vi "Startup.vi"(8 "Error In":errorcluster) -> (0 "Error Out":errorcluster)   [LabVIEW 2018]
uses:
  <vilib>/Utility/miscctls.llb/LVPointTypeDef.ctl
  Libraries/Tracker Main/Tracker Main.lvlib
panel:
  in  "Tracker Main to start":bool
  out "Status":string
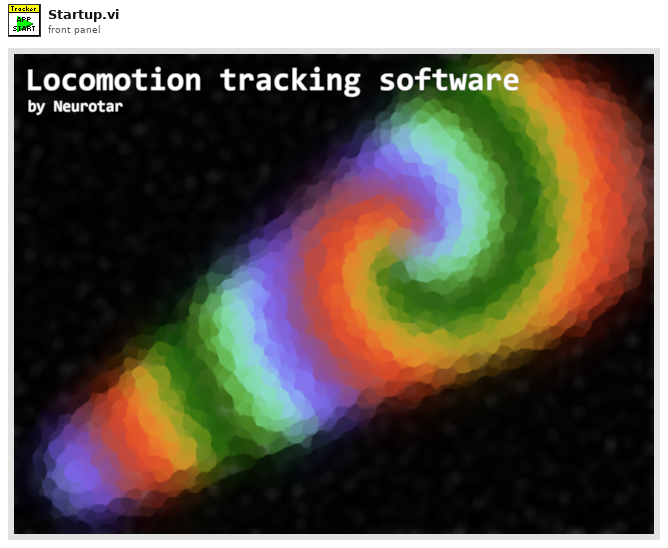
[diagram p1: front panel]
types:
  T1 = typedef "LVPointTypeDef.ctl" = cluster{"Horizontal":i16, "Vertical":i16}
  T2 = enum32{"Invalid", "Standard", "Closed", "Hidden", "Minimized", "Maximized"}
  T3 = typedef "Tracker Main.lvlib/Broadcast Events--cluster.ctl" = cluster{"Module Did Init":refnum<user-event>, "Status Updated":refnum<user-event>, "Error Reported":refnum<user-event>, "Module Did Stop":refnum<user-event>, "Update Module Execution Status":refnum<user-event>}
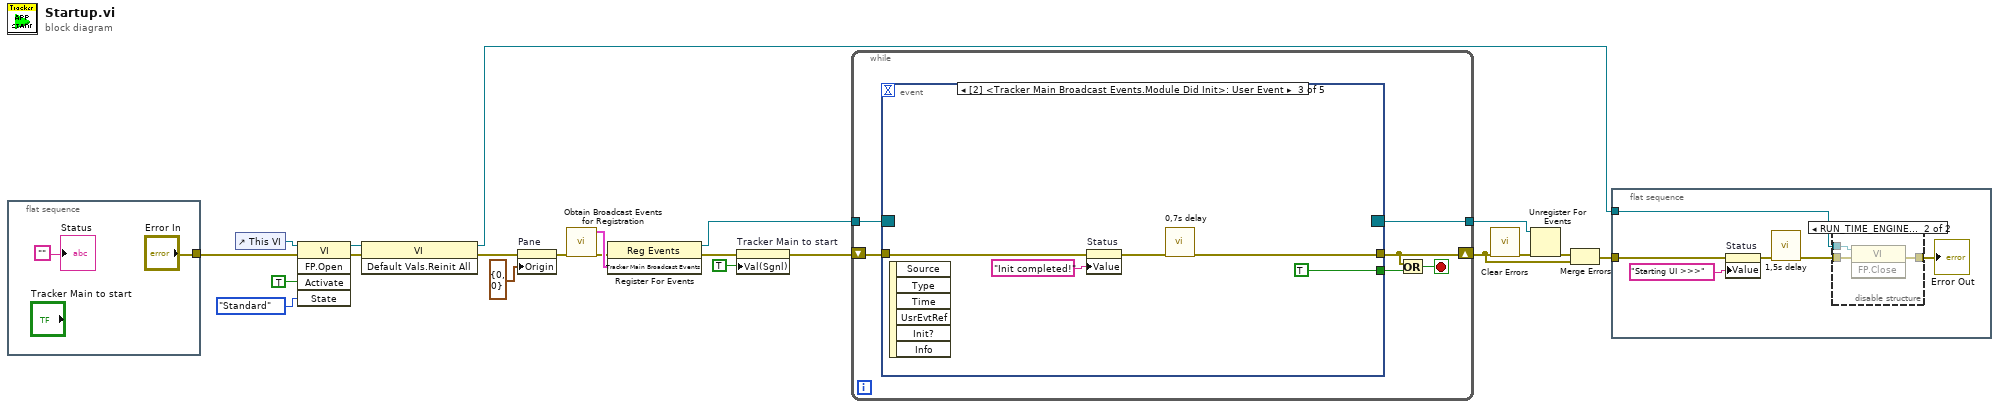
[diagram p0: block diagram]
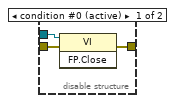
[diagram p2: hidden frame]
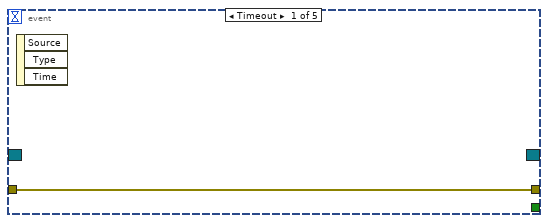
[diagram p3: hidden frame]
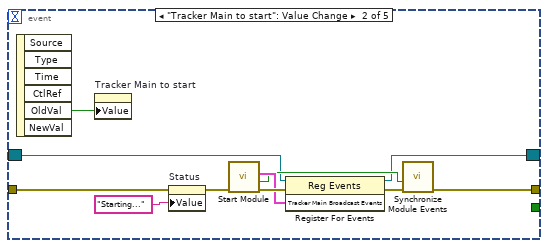
[diagram p4: hidden frame]
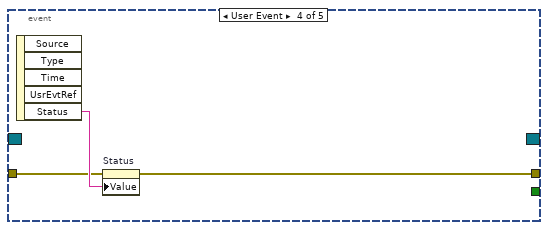
[diagram p5: hidden frame]
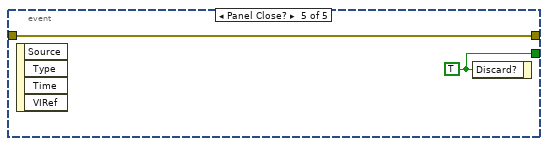
[diagram p6: hidden frame]
diagram:
  n1 = flat-sequence {
    tunnel: ["Error In"] -> w20
    frame #0 {
      "Status" <- ""
    }
  }
  n2 = control-ref of="This VI"() -> (w21:refnum<vi>)
  n3 = invoke class="VI" method="FP.Open"(reference=w21, error in=w20, "Activate"=TRUE ("Activate?"), "State"=T2."Standard") -> (reference out=w16:refnum<vi>, error out=w17:errorcluster)  [unwired: 1 in, 3 out]
  n4 = invoke class="VI" method="Default Vals.Reinit All"(reference=w16, error in=w17) -> (reference out=w1:refnum<vi>, error out=w15:errorcluster)  [unwired: 1 in, 1 out]
  n5 = property on="Pane" class="Pane"(error in=w15, "Origin"=T1 {"Horizontal"=0, "Vertical"=0}) -> (error out=w7:errorcluster)  [unwired: 1 in, 1 out]
  n6 = call "Obtain Broadcast Events for Registration.vi"("error in (no error)"=w7) -> ("error out"=w12:errorcluster, "Tracker Main Broadcast Events"=w13:T3)  [unwired: 8 in, 1 out]
  n7 = register-events(error in=w12, w13) -> (reference out=w11:refnum<event-registration>, error out=w10:errorcluster)  [unwired: 1 in]
  n8 = property on="Tracker Main to start" class="Bool (strict)"(error in=w10, "Val(Sgnl)"=TRUE ("Value (Signaling)")) -> (error out=w9:errorcluster)  [unwired: 1 in, 1 out]
  n9 = while {
    tunnel: w11 -> [w29]
    shift-right: [w25] -> w6
    shift-left: w9 -> [w28]
    tunnel: [w24] -> w3
    stop <- w26 stop-if-true
    n10 = event shown="[2] <Tracker Main Broadcast Events.Module Did Init>: User Event" {
      selector: w29 -> [_ w37 _ _ _]
      dyn-events: [_ w36 _ _ _] -> w24
      timeout: _ -> [_ _ _ _ _]
      tunnel: w28 -> [w30 w32 w45 w48 w50]
      tunnel: [w30 w35 w42 w47 w50] -> w25
      tunnel: [_ _ TRUE _ w51] -> w27
      event Timeout {
        n11 = event-data() -> ()  [unwired: 1 in, 3 out]
      }
      event "Tracker Main to start": Value Change {
        n12 = event-data() -> ("OldVal"=w34:bool)  [unwired: 1 in, 5 out]
        n13 = property on="Tracker Main to start" class="Bool (strict)"("Value"=w34) -> ()  [unwired: 2 in, 2 out]
        n14 = property on="Status" class="Str"(error in=w32, "Value"="Starting..." ("Status")) -> (error out=w31:errorcluster)  [unwired: 1 in, 1 out]
        n15 = call "Start Module.vi"("error in (no error)"=w31) -> ("error out"=w41:errorcluster, "Wait for Event Sync?"=w38:bool, "Tracker Main Broadcast Events"=w40:T3)  [unwired: 7 in, 1 out]
        n16 = register-events(reference=w37, error in=w41, w40) -> (reference out=w36:refnum<event-registration>, error out=w39:errorcluster)
        n17 = call "Synchronize Module Events.vi"("error in (no error)"=w39, "Wait for Event Sync?"=w38) -> ("error out"=w35:errorcluster)  [unwired: 9 in]
      }
      event User Event {
        n18 = event-data() -> ()  [unwired: 1 in, 6 out]
        n19 = property on="Status" class="Str"(error in=w45, "Value"="Init completed!" ("Status")) -> (error out=w43:errorcluster)  [unwired: 1 in, 1 out]
        n20 = call "0,7s delay"("error in (no error)"=w43) -> ("error out"=w42:errorcluster)  [unwired: 10 in]
      }
      event User Event {
        n21 = event-data() -> ("Status"=w49:string)  [unwired: 1 in, 4 out]
        n22 = property on="Status" class="Str"(error in=w48, "Value"=w49) -> (error out=w47:errorcluster)  [unwired: 1 in, 1 out]
      }
      event Panel Close? {
        w51 = TRUE ("Discard?")
        n23 = event-data() -> ()  [unwired: 1 in, 4 out]
        n24 = event-data("Discard?"=w51) -> ()  [unwired: 1 in, 1 out]
      }
    }
    n25 = Or(x=w25, y=w27) -> (x .or. y?=w26:bool)
  }
  n26 = call <vilib>:"Clear Errors.vi"("error in (no error)"=w6) -> ("error out"=w4:errorcluster)  [unwired: 5 in, 1 out]
  n27 = Unregister For Events(event registration refnum=w3, error in=w4) -> (error out=w5:errorcluster)
  n28 = Merge Errors(w5, w6) -> (w2:errorcluster)
  n29 = flat-sequence {
    tunnel: w2 -> [w55]
    tunnel: w1 -> [w57]
    frame #0 {
      n30 = property on="Status" class="Str"(error in=w55, "Value"="Starting UI >>>" ("Status")) -> (error out=w54:errorcluster)  [unwired: 1 in, 1 out]
      n31 = call "1,5s delay"("error in (no error)"=w54) -> ("error out"=w53:errorcluster)  [unwired: 10 in]
      n32 = disable-structure shown="RUN_TIME_ENGINE==True" {
        disable-tunnel: w57 -> [w60 w63]
        disable-tunnel: w53 -> [w59 w62]
        disable-tunnel: [w58 w61] -> w52
        frame condition #0 (active) {
          n33 = invoke class="VI" method="FP.Close"(reference=w60, error in=w59) -> (error out=w58:errorcluster)  [unwired: 1 in, 2 out]
        }
        frame condition #1 {
          n34 = invoke class="VI" method="FP.Close"(reference=w63, error in=w62) -> (error out=w61:errorcluster)  [unwired: 1 in, 2 out]
        }
      }
      "Error Out" <- w52
    }
  }
